vi "Get Icon Class from Data.vi"(8 "error in (no error)":errorcluster, 9 "BW Icon":T1, 10 "Color Icon":T1, 11 "Icon Data":T2={"Text Visible?"=FALSE, "Text Opacity"=0, "Templ Visible?"=FALSE, "Templ Opacity"=0, "Relative Path from 1 to 2"=path "", "Image"=bytes[0], "All User Layers"=[], "Body Text"={"Line 1 text"="", "Line 2 text"="", "Line 3 text"="", "Line 4 text"="", "Line 1 color"=0, "Line 2 color"=0, "Line 3 color"=0, "Line 4 color"=0, "Body Text Spec"={"Font"="", "Alignment"=0, "Size"=3}, "Center text vertically"=FALSE, "Capitalize Text"=FALSE}} {"Body Text"."Body Text Spec"."Alignment" items=["left", "center", "right"]}) -> (0 "error out":errorcluster, 3 "Icon out":refnum<class "Icon.lvclass">)   [LabVIEW 2021, in "LabVIEW Icon API.lvlib"]
doc: "Generate Icon class from the passed in data."
uses:
  LabVIEW Icon API.lvlib
  <vilib>/picture/picture.llb/imagedata.ctl
  lv_icon/Classes/Icon/Icon.lvclass
  lv_icon/Controls/LabVIEW Icon Stored Information.ctl
  lv_icon/Classes/Layer/Layer.lvclass
  lv_icon/Controls/BodyText.ctl
  lv_icon/Controls/Font.ctl
  lv_icon/Controls/Alignment.ctl
panel:
  in  "Localied string text":string="Text"
  in  "Localized string template":string="Template"
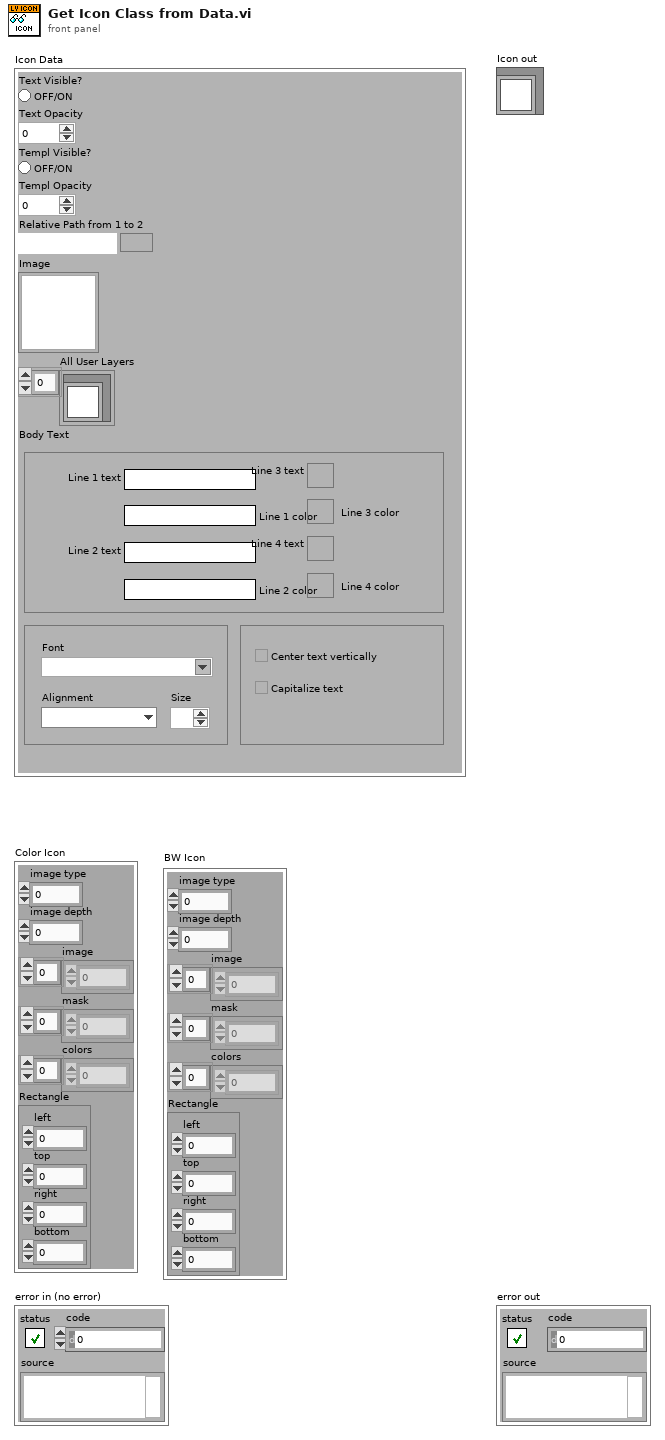
[diagram p1: front panel]
types:
  T1 = typedef "imagedata.ctl" = cluster{"image type":i32, "image depth":i32, "image":u8[], "mask":u8[], "colors":u32[], "Rectangle":cluster{"left":i16, "top":i16, "right":i16, "bottom":i16}}
  T2 = typedef "LabVIEW Icon Stored Information.ctl" = cluster{"Text Visible?":bool, "Text Opacity":u8, "Templ Visible?":bool, "Templ Opacity":u8, "Relative Path from 1 to 2":path, "Image":picture, "All User Layers":refnum<class "Layer.lvclass">[], "Body Text":T3}
  T3 = typedef "BodyText.ctl" = cluster{"Line 1 text":string, "Line 2 text":string, "Line 3 text":string, "Line 4 text":string, "Line 1 color":u32, "Line 2 color":u32, "Line 3 color":u32, "Line 4 color":u32, "Body Text Spec":cluster{"Font":T4, "Alignment":T5, "Size":u8}, "Center text vertically":bool, "Capitalize Text":bool}
  T4 = typedef "Font.ctl" = string
  T5 = typedef "Alignment.ctl" = u16
  T6 = typedef "Layer.ctl" = cluster{"LayerIcon":picture, "LayerName":string, "Opacity":u8, "Visibility?":bool}
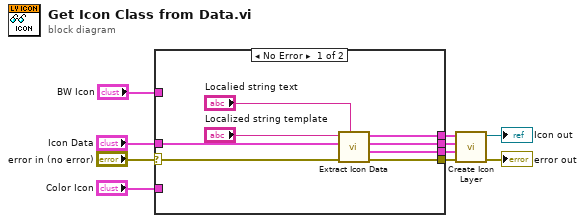
[diagram p0: block diagram]
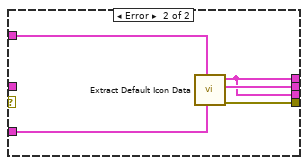
[diagram p2: hidden frame]
diagram:
  n1 = case shown="No Error" "error in (no error)" {
    selector: "error in (no error)" -> [w17 _]
    tunnel: [w17 w21] -> w7
    tunnel: "Icon Data" -> [w16 _]
    tunnel: [w14 w19] -> w4
    tunnel: [w13 w22] -> w5
    tunnel: [w12 w19] -> w6
    tunnel: "Color Icon" -> [_ w20]
    tunnel: "BW Icon" -> [_ w18]
    frame No Error {
      n2 = call "Extract Icon Data.vi"("Text layer name"="Localied string text", "Icon data in"=w16, "Template layer name"="Localized string template") -> ("Template data"=w12:T6, "Icon data out"=w13:T2, "Text data"=w14:T6)  [unwired: 5 in, 1 out]
    }
    frame Error {
      n3 = call "Extract Default Icon Data.vi"("Color Icon"=w20, "BW Icon"=w18) -> ("error out"=w21:errorcluster, "VI Icon Data out"=w22:T2, "Default Icon Template data"=w19:T6)  [unwired: 7 in]
    }
  }
  n4 = call "Create Icon Layer.vi"("error in (no error)"=w7, "Template data"=w6, "Icon data"=w5, "Text data"=w4) -> ("error out"=→"error out":errorcluster, "Icon out"=→"Icon out":refnum<class "Icon.lvclass">)  [unwired: 6 in]
